vi "Server Subscription.vi"(6 "Active (T)":bool=TRUE, 7 "UpdateRate (1000)":i32=1000, 8 "error in (no error)":errorcluster, 10 "Name":string="MySubsription", 11 ".NET Refnum in":refnum<k24>) -> (0 "error out":errorcluster, 2 "CreateSubscription":refnum<k24>, 3 ".NET Refnum out":refnum<k24>)   [LabVIEW 2024, in "LV_OPC_NET.lvlib"]
uses:
  LV_OPC_NET.lvlib
  C:/Users/108003658/OneDrive - Baker Hughes/Desktop/LV_OPC-Client-x64/LV_OPC_Test/OPC.NET/OpcNetApi.dll
  OpcNetApi.dll
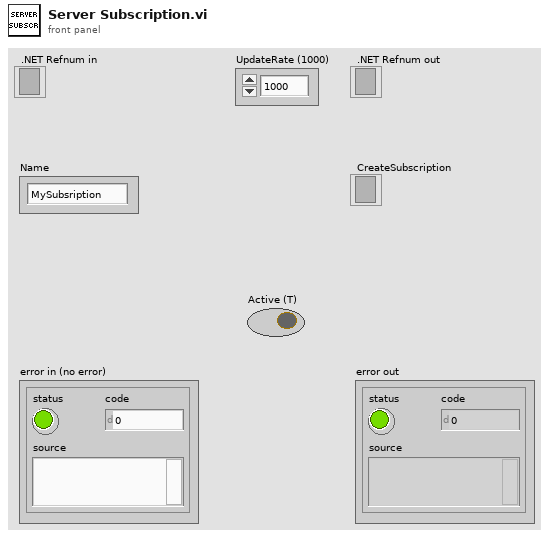
[diagram p1: front panel]
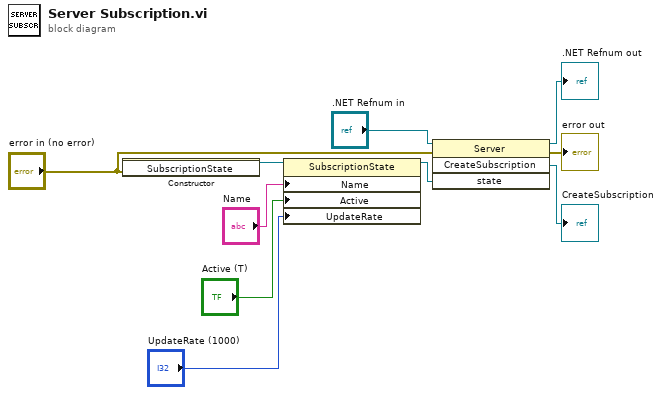
[diagram p0: block diagram]
diagram:
  n1 = constructor class="SubscriptionState"(error in="error in (no error)") -> (reference out=w1:refnum<k24>)  [unwired: 2 in, 2 out]
  n2 = property class="SubscriptionState"(reference=w1, "Name"="Name", "Active"="Active (T)", "UpdateRate"="UpdateRate (1000)") -> (reference out=w5:refnum<k24>)  [unwired: 1 in, 1 out]
  n3 = invoke class="Server" method="CreateSubscription"(reference=".NET Refnum in", error in="error in (no error)", "state"=w5) -> (reference out=→".NET Refnum out":refnum<k24>, error out=→"error out":errorcluster, "CreateSubscription"=→"CreateSubscription":refnum<k24>)  [unwired: 1 in, 1 out]
